vi "习题4.4.vi"() -> ()   [LabVIEW 2017]
panel:
  out "布尔":bool
  in  "滑动杆":dbl(slide) scale=-50.0..50.0
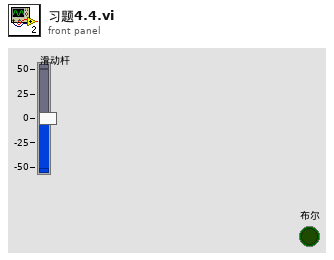
[diagram p1: front panel]
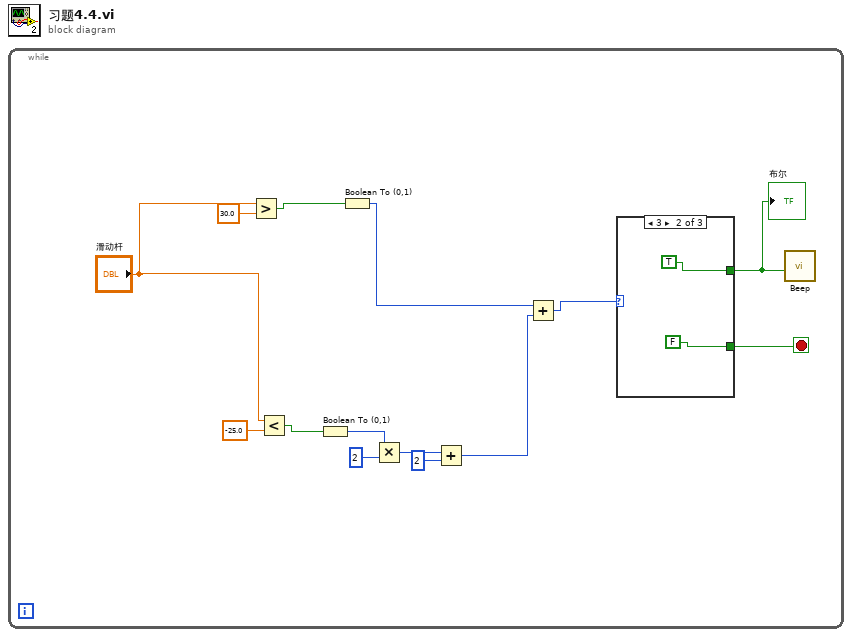
[diagram p0: block diagram]
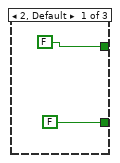
[diagram p2: hidden frame]
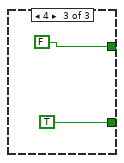
[diagram p3: hidden frame]
diagram:
  n1 = while {
    stop <- w2 stop-if-true
    n2 = Greater?(x="滑动杆", y=30.0) -> (0:w6:bool)
    n3 = Less?(x="滑动杆", y=-25.0) -> (x < y?=w11:bool)
    n4 = Boolean To (0,1)(Boolean=w11) -> (0, 1=w10:i16)
    n5 = Boolean To (0,1)(Boolean=w6) -> (0, 1=w5:i16)
    n6 = Multiply(x=w10, y=i16 2) -> (x*y=w9:i16)
    n7 = Add(x=w9, y=i16 2) -> (x+y=w4:i16)
    n8 = Add(x=w5, y=w4) -> (x+y=w3:i16)
    n9 = case shown="3" w3 {
      tunnel: [FALSE TRUE FALSE] -> w1
      tunnel: [FALSE FALSE TRUE] -> w2
      frame 2, Default {
      }
      frame 3 {
      }
      frame 4 {
      }
    }
    "布尔" <- w1
    n10 = call <vilib>:"Beep.vi"("use system alert? (T)"=w1) -> ()  [unwired: 11 in]
  }
